vi "Interrupt Notifier.vi"(8 "error in":errorcluster) -> (0 "error out":errorcluster, 3 "Notifier out":refnum<notifier>)   [LabVIEW 2013, in "LVTM.lvlib"]
uses:
  LVTM.lvlib
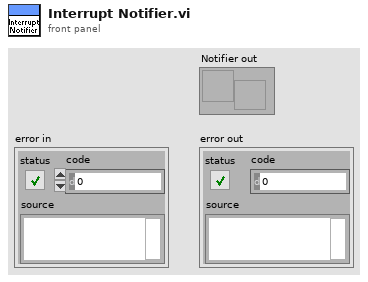
[diagram p1: front panel]
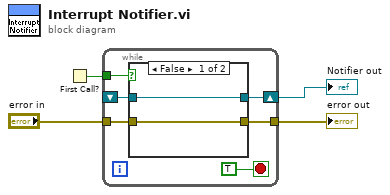
[diagram p0: block diagram]
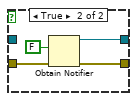
[diagram p2: hidden frame]
diagram:
  n1 = First Call?() -> (First Call?: T/F=w1:bool)
  n2 = while {
    tunnel: w1 -> [w9]
    shift-right: [w8] -> w4
    shift-left: _ -> [w5]
    tunnel: "error in" -> [w7]
    tunnel: [w6] -> w3
    stop <- TRUE stop-if-true
    n3 = case shown="False" w9 {
      tunnel: [w12 w15] -> w8
      tunnel: w7 -> [w11 w14]
      tunnel: [w11 w13] -> w6
      tunnel: w5 -> [w12 _]
      frame False {
      }
      frame True {
        n4 = Obtain Notifier(notification data type=FALSE, error in (no error)=w14) -> (notifier out=w15:refnum<notifier>, error out=w13:errorcluster)  [unwired: 2 in, 1 out]
      }
    }
  }
  "Notifier out" <- w4
  "error out" <- w3
